vi "write_params.vi"(8 "error in (no error)":errorcluster caption="entrée d'erreur (pas d'erreur)", 10 "params":T1={"fit_intercept"=TRUE, "verbose"={"verbose_type"="bool", "verbose_bool"=FALSE, "verbose_int"=0.0}, "normalize"=TRUE, "precompute"={"precompute_type"="auto", "precompute_bool"=FALSE, "precompute_list"=[]}, "n_nonzero_coefs"=500.0, "eps"=1e-07, "copy_X"=TRUE, "fit_path"=TRUE, "jitter"={"jitter_type"="None", "jitter_float"=0.0}, "random_state"=0.0}, 11 "Lars en entrée":refnum<class "Lars.lvclass">) -> (0 "error out":errorcluster caption="sortie d'erreur", 3 "Lars en sortie":refnum<class "Lars.lvclass">)   [LabVIEW 2020, in "Lars.lvclass"]
uses:
  Lars.lvclass
  Controls/lars_params.ctl
  Lars.lvclass/Lars.ctl
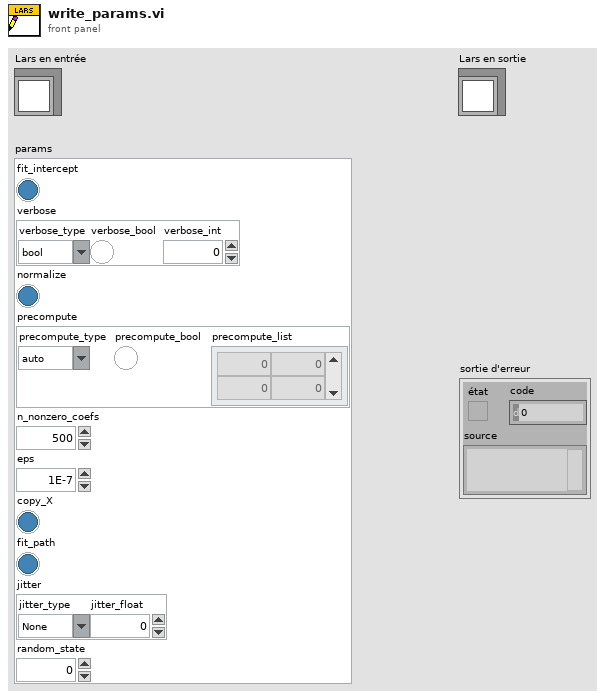
[diagram p1: front panel]
types:
  T1 = typedef "lars_params.ctl" = cluster{"fit_intercept":bool, "verbose":cluster{"verbose_type":string, "verbose_bool":bool, "verbose_int":dbl}, "normalize":bool, "precompute":cluster{"precompute_type":string, "precompute_bool":bool, "precompute_list":dbl[][]}, "n_nonzero_coefs":dbl, "eps":dbl, "copy_X":bool, "fit_path":bool, "jitter":cluster{"jitter_type":string, "jitter_float":dbl}, "random_state":dbl}
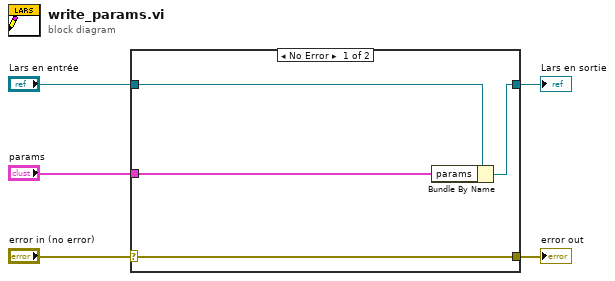
[diagram p0: block diagram]
diagram:
  n1 = case shown="No Error" "error in (no error)" {
    selector: "error in (no error)" -> [w9 w10]
    tunnel: [w9 w10] -> w4
    tunnel: [w7 w11] -> w2
    tunnel: "Lars en entrée" -> [w8 w11]
    tunnel: "params" -> [w6 _]
    frame No Error {
      n2 = Bundle By Name(cluster=w8, "params"=w6) -> (w7:refnum<class "Lars.lvclass">)
    }
    frame Error {
    }
  }
  "error out" <- w4
  "Lars en sortie" <- w2
